vi "Read.vi"(8 "error in (no error)":errorcluster, 11 "IVI Oscilloscope in":refnum<class "IVI Oscilloscope.lvclass">) -> (0 "error out":errorcluster, 1 "timed out?":bool, 2 "Data":refnum<class "AbstractData.lvclass">, 3 "IVI Oscilloscope out":refnum<class "IVI Oscilloscope.lvclass">)   [LabVIEW 2014, in "IVI Oscilloscope.lvclass"]
uses:
  IVI Oscilloscope.lvclass
  Framework/Model/Data/AbstractData/AbstractData.lvclass
  IVI Oscilloscope.lvclass/IVI Oscilloscope.ctl
  Framework/Model/Data/Data1D/Data1D.lvclass
  Framework/Interfaces/Observable Actor/Observable Actor.lvclass
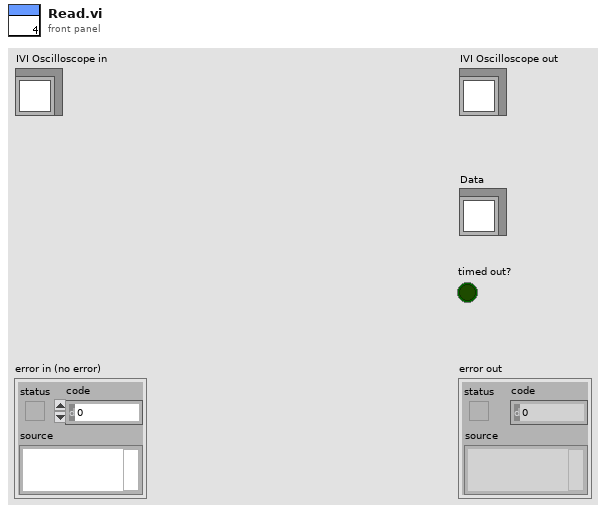
[diagram p1: front panel]
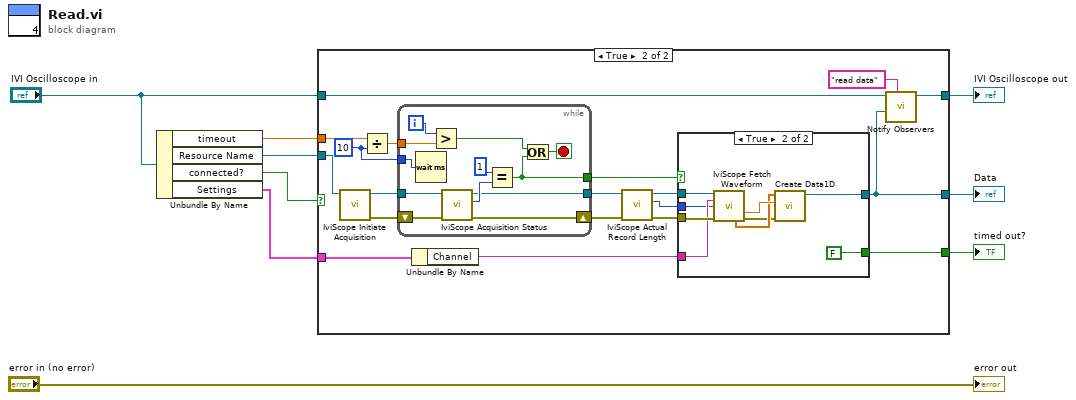
[diagram p0: block diagram]
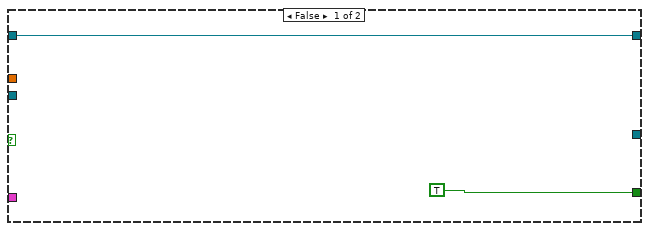
[diagram p2: hidden frame]
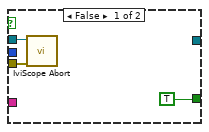
[diagram p3: hidden frame]
diagram:
  n1 = Unbundle By Name("IVI Oscilloscope in") -> ("timeout"=w4:dbl, "Resource Name"=w6:refnum<k15>, "connected?"=w7:bool, "Settings"=w2:cluster{"Channel":string})
  n2 = case shown="True" w7 {
    tunnel: "IVI Oscilloscope in" -> [w11 w19]
    tunnel: [w11 w18] -> w8
    tunnel: w6 -> [_ w30]
    tunnel: [_ w16] -> w5
    tunnel: w4 -> [_ w20]
    tunnel: w2 -> [_ w28]
    tunnel: [TRUE w26] -> w1
    frame False {
    }
    frame True {
      w13 = u32 10 ("y")
      n3 = call <vilib>:"IviScope Initiate Acquisition.vi"("instrument handle"=w30) -> ("error out"=w15:errorcluster, "instrument handle out"=w29:refnum<k15>)  [unwired: 9 in]
      n4 = Divide(x=w20, y=w13) -> (x/y=w14:dbl)
      n5 = while {
        tunnel: w14 -> [w37]
        tunnel: w13 -> [w34]
        tunnel: w29 -> [w42]
        tunnel: [w40] -> w25
        shift-right: [w39] -> w24
        shift-left: w15 -> [w38]
        tunnel: [w31] -> w12
        i -> [w36]
        stop <- w33 stop-if-true
        n6 = Wait (ms)(milliseconds to wait=w34) -> ()  [unwired: 1 out]
        n7 = Greater?(x=w36, y=w37) -> (0:w32:bool)
        n8 = call <vilib>:"IviScope Acquisition Status.vi"("error in (no error)"=w38, "instrument handle"=w42) -> ("error out"=w39:errorcluster, "acquisition status"=w41:i32, "instrument handle out"=w40:refnum<k15>)  [unwired: 7 in]
        n9 = Equal?(x=1, y=w41) -> (x = y?=w31:bool)
        n10 = Or(x=w32, y=w31) -> (x .or. y?=w33:bool)
      }
      n11 = Unbundle By Name(w28) -> ("Channel"=w27:string)
      n12 = call <vilib>:"IviScope Actual Record Length.vi"("error in (no error)"=w24, "instrument handle"=w25) -> ("error out"=w22:errorcluster, "actual record length"=w21:i32, "instrument handle out"=w23:refnum<k15>)  [unwired: 7 in]
      n13 = case shown="True" w12 {
        tunnel: w23 -> [w45 w54]
        tunnel: w22 -> [w44 w53]
        tunnel: w27 -> [_ w52]
        tunnel: [_ w49] -> w16
        tunnel: [TRUE FALSE] -> w26
        tunnel: w21 -> [_ w47]
        frame False {
          n14 = call <vilib>:"IviScope Abort.vi"("error in (no error)"=w44, "instrument handle"=w45) -> ()  [unwired: 8 in, 2 out]
        }
        frame True {
          n15 = call <vilib>:"IviScope Fetch Waveform.vi"("instrument handle"=w54, "channel name (\"CHANNEL1\")"=w52, "waveform size (0)"=w47, "error in (no error)"=w53) -> ("x increment"=w51:dbl, "waveform array"=w50:dbl[], "error out"=w46:errorcluster)  [unwired: 6 in, 3 out]
          n16 = call "Create Data1D.vi"("error in (no error)"=w46, "dt"=w51, "Array"=w50) -> ("Data1D out"=w49:refnum<class "Data1D.lvclass">)  [unwired: 7 in, 1 out]
        }
      }
      n17 = call "Notify Observers.vi"("name"="read data", "value"=w16, "Observable Actor in"=w19) -> ("Observable Actor out"=w18:refnum<class "IVI Oscilloscope.lvclass">)  [unwired: 7 in, 1 out]
    }
  }
  "IVI Oscilloscope out" <- w8
  "Data" <- w5
  "timed out?" <- w1
  "error out" <- "error in (no error)"
